vi "Initialize.vi"(8 "error in (no error)":errorcluster, 10 "Namespace Delimiter":string(combo)=":") -> (0 "error out":errorcluster)   [LabVIEW 2020, in "Tag Engine.lvlib"]
doc: "Initialize the Tag store.\n\nCall this VI at the startup of your main process (that does not leave memory until your application is stopped). The Tag store will be owned by this process."
uses:
  Tag Engine.lvlib
  Core/Tag Core.lvclass
panel:
  # "Default delimiter is \":'\nBut you could use \"::\"\nor \"_\""
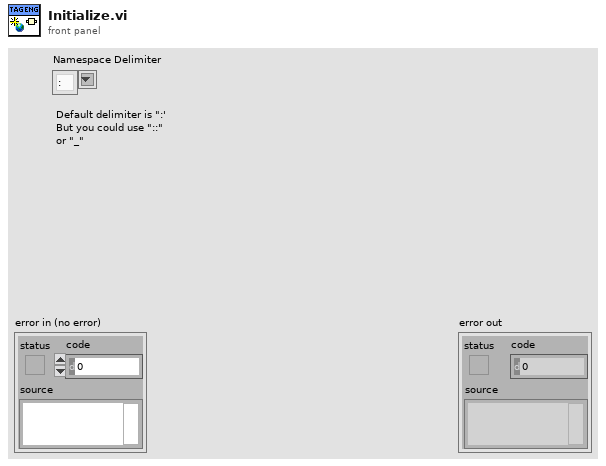
[diagram p1: front panel]
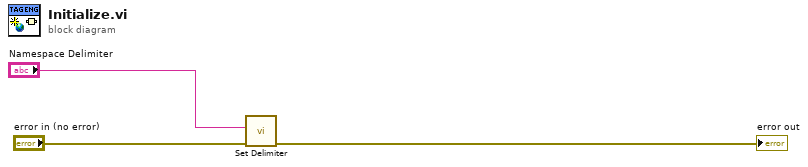
[diagram p0: block diagram]
diagram:
  n1 = call "Set Delimiter.vi"("error in (no error)"="error in (no error)", "Namespace Delimiter"="Namespace Delimiter") -> ("error out"=→"error out":errorcluster)  [unwired: 9 in]
